vi "Create Image.vi"   [LabVIEW 2020, in "g_ar_toolkit.image.lvlib"]
doc: "Create an empty image. \n\nsSpecify the size if you need to preallocate the memory for EDVR based operations."
uses:
  g_ar_toolkit.image.lvlib
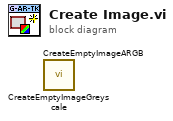
[diagram p0: block diagram]
diagram:
  n1 = call "CreateEmptyImageGreyscale.vi"() -> ()  [unwired: 10 in, 2 out]
  n2 = call "CreateEmptyImageARGB.vi"() -> ()  [unwired: 10 in, 2 out]
